vi "Write Table Configuration.vi"(8 "error in (no error)":errorcluster, 10 "Table Configuration":refnum<class "Table Configuration Interface.lvclass">, 11 "Basic Table in":refnum<class "Basic Table.lvclass">) -> (0 "error out":errorcluster, 3 "Basic Table out":refnum<class "Basic Table.lvclass">)   [LabVIEW 2020]
uses:
  Basic Table.lvclass
  Table Configuration Interface/Table Configuration Interface.lvclass
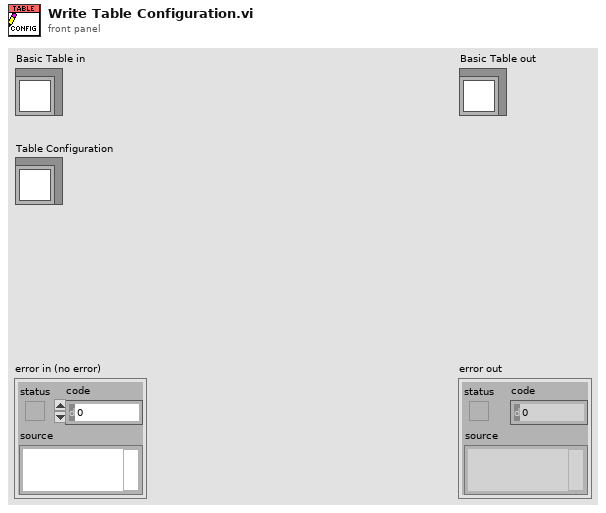
[diagram p1: front panel]
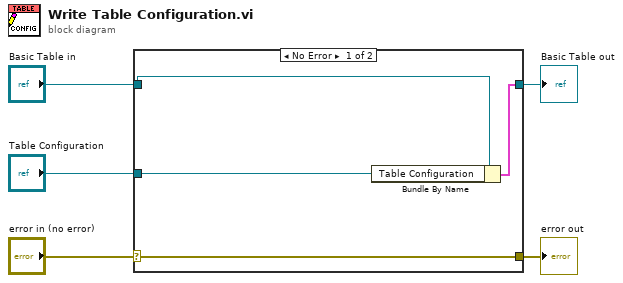
[diagram p0: block diagram]
diagram:
  n1 = case shown="No Error" "error in (no error)" {
    selector: "error in (no error)" -> [w9 w10]
    tunnel: [w9 w10] -> w4
    tunnel: [w7 w11] -> w2
    tunnel: "Basic Table in" -> [w8 w11]
    tunnel: "Table Configuration" -> [w6 _]
    frame No Error {
      n2 = Bundle By Name(cluster=w8, "Table Configuration"=w6) -> (w7:cluster{})
    }
    frame Error {
    }
  }
  "error out" <- w4
  "Basic Table out" <- w2
